vi "caraya test runner.vi"() -> ()   [LabVIEW 2024]
uses:
  <vilib>/addons/_JKI Toolkits/Caraya/classes/Test Report.JUnit/Test Report.JUnit.lvclass
  C:/Program Files/National Instruments/LabVIEW 2024/vi.lib/addons/_JKI Toolkits/Caraya/classes/Test Report/Test Report.lvclass
  <vilib>/addons/_JKI Toolkits/Caraya/classes/Test Runner.Folder/Test Runner.Folder.lvclass
  C:/Program Files/National Instruments/LabVIEW 2024/vi.lib/addons/_JKI Toolkits/Caraya/classes/Test Runner/Test Runner.lvclass
  <vilib>/addons/_JKI Toolkits/Caraya/classes/Test Runner/Test Runner.lvclass
panel:
  out "error out":errorcluster
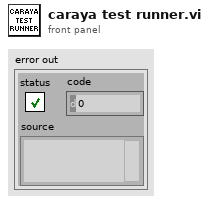
[diagram p1: front panel]
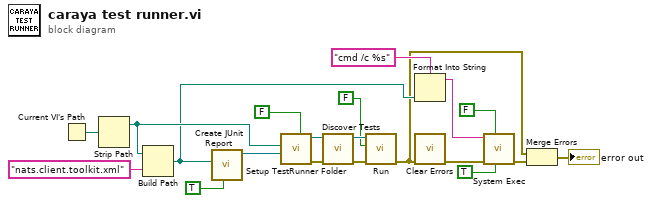
[diagram p0: block diagram]
diagram:
  n1 = Current VI's Path() -> (path=w17:path)
  n2 = Strip Path(path=w17) -> (stripped path=w10:path)  [unwired: 1 out]
  n3 = Build Path(base path=w10, name or relative path="nats.client.toolkit.xml") -> (appended path=w8:path)
  n4 = call <vilib>:"Create JUnit Report.vi"("Verbose"=TRUE, "Report Path"=w8) -> ("Test Report.JUnit out"=w15:refnum<class "Test Report.JUnit.lvclass">)  [unwired: 8 in, 1 out]
  n5 = call <vilib>:"Setup TestRunner Folder.vi"("Interactive (T)"=FALSE, "Test Report"=w15, "Directory to search"=w10) -> ("error out"=w12:errorcluster, "Test Runner.Folder out"=w14:refnum<class "Test Runner.Folder.lvclass">)  [unwired: 7 in]
  n6 = call <vilib>:"Discover Tests.vi"("error in (no error)"=w12, "Test Runner in"=w14) -> ("error out"=w18:errorcluster, "Test Runner out"=w20:refnum<class "Test Runner.Folder.lvclass">)  [unwired: 8 in]
  n7 = call <vilib>:"Run.vi"("error in (no error)"=w18, "Interactive"=FALSE, "Test Runner in"=w20) -> ("error out"=w3:errorcluster)  [unwired: 6 in, 2 out]
  n8 = Format Into String(format string="cmd /c %s", w8) -> (resulting string=w7:string)  [unwired: 2 in, 1 out]
  n9 = call <vilib>:"Clear Errors.vi"("error in (no error)"=w3) -> ("error out"=w2:errorcluster)  [unwired: 5 in, 1 out]
  n10 = call <vilib>:"System Exec.vi"("run minimized? (F)"=TRUE, "wait until completion? (T)"=FALSE, "error in (no error)"=w2, "command line"=w7) -> ("error out"=w5:errorcluster)  [unwired: 4 in, 3 out]
  n11 = Merge Errors(w3, w5) -> (→"error out":errorcluster)
